vi "Update Nested State.vi"(8 "error in (no error)":errorcluster, 10 "Module Status":T1, 11 "Module in":refnum<class "Module.lvclass">) -> (0 "error out":errorcluster, 3 "Module out":refnum<class "Module.lvclass">)   [LabVIEW 2020, in "Volatus.lvlib" / "Module.lvclass"]
uses:
  Module.lvclass
  Module Status Update.ctl
  MessageQ/MessageQ.lvclass
  State.ctl
  Module.lvclass/Module.ctl
  Volatus.lvlib
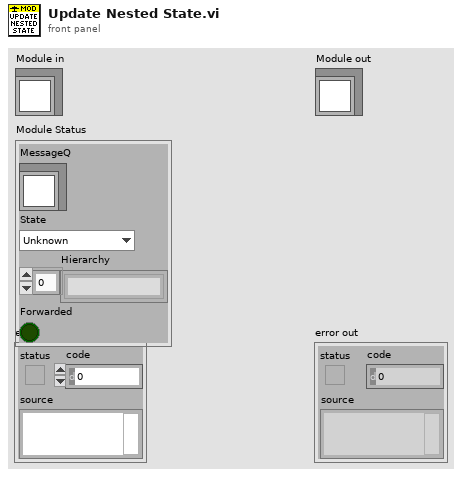
[diagram p1: front panel]
types:
  T1 = typedef "Volatus.lvlib/Module Status Update.ctl" = cluster{"MessageQ":refnum<class "MessageQ.lvclass">, "State":T2, "Hierarchy":string[], "Forwarded":bool}
  T2 = typedef "Volatus.lvlib/Module.lvclass/State.ctl" = enum16{"Unknown", "Launched", "Starting", "Running", "Stopping", "Stopped", "Error - Starting", "Error - Run", "Error - Stopping"}
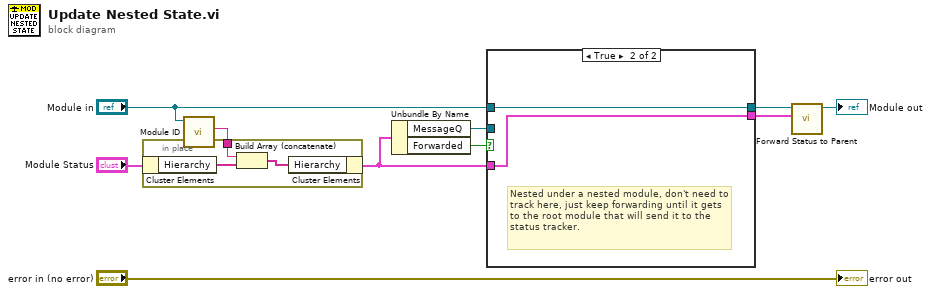
[diagram p0: block diagram]
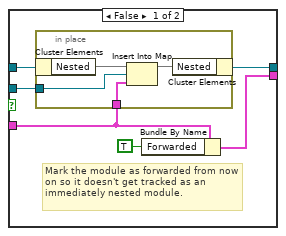
[diagram p2: hidden frame]
diagram:
  n1 = call-dynamic "Module ID.vi"("Module in"="Module in") -> ("Module ID"=w5:string)  [unwired: 10 in]
  n2 = in-place {
    in-place-border: w5 -> [w11]
    n3 = in-place-cluster #1("Module Status") -> ("Hierarchy"=w13:string[])
    n4 = Build Array (concatenate)(w11, w13) -> (w12:string[])
    n5 = in-place-cluster #1("Hierarchy"=w12) -> (w3:T1)
  }
  n6 = Unbundle By Name(w3) -> ("MessageQ"=w8:refnum<class "MessageQ.lvclass">, "Forwarded"=w1:bool)
  n7 = case shown="True" w1 {
    tunnel: [w19 w25] -> w9
    tunnel: w8 -> [w18 _]
    tunnel: "Module in" -> [w17 w25]
    tunnel: w3 -> [w16 w24]
    tunnel: [w15 w24] -> w2
    frame False {
      # "Mark the module as forwarded from now on so it doesn't get tracked as an immediately nested module."
      n8 = in-place {
        in-place-border: w18 -> [w21]
        in-place-border: w16 -> [w22]
        n9 = in-place-cluster #2(w17) -> ("Nested"=w23:map{refnum<class "MessageQ.lvclass">, T1})
        n10 = Insert Into Map(map in=w23, key=w21, value=w22) -> (map out=w20:map{refnum<class "MessageQ.lvclass">, T1})  [unwired: 2 out]
        n11 = in-place-cluster #2("Nested"=w20) -> (w19:refnum<class "Module.lvclass">)
      }
      n12 = Bundle By Name(cluster=w16, "Forwarded"=TRUE) -> (w15:T1)
    }
    frame True {
      # "Nested under a nested module, don't need to track here, just keep forwarding until it gets to the root module that will send it to the status tracker."
    }
  }
  n13 = call "Forward Status to Parent.vi"("Module Status"=w2, "Module in"=w9) -> ("Module out"=→"Module out":refnum<class "Module.lvclass">)  [unwired: 8 in, 1 out]
  "error out" <- "error in (no error)"
